vi "Remap Controls.vi"   [LabVIEW 2015]
uses:
  Common Code/Driver Control Selector.ctl
  Common Code/Manipulator Control Selector.ctl
  <vilib>/Rock Robotics/WPI/Utilities/WPI_GetSetVariantRefNum.vi
  Robot Global Data.vi
types:
  T1 = typedef "Manipulator Control Selector.ctl" = enum16{"High Pressure Shot", "Manual Climb Mode", "Auto Climb Mode", "Eject", "Intake", "Manual/Auto Toggle", "Re-seat", "Intake Down", "None"}
  T2 = typedef "Driver Control Selector.ctl" = enum16{"Creep Up", "Creep Down", "Creep Left", "Creep Right", "Forward/Backward", "Right/Left", "Outer Shot", "Batter Shot", "Shoot", "Climb", "Flashlight", "None"}
  T3 = typedef "Manipulator Control Remap.ctl" = cluster{"High Pressure Shot (B)":bool, "Manual Climb Mode (B)":bool, "Auto Climb Mode (B)":bool, "Eject (B)":bool, "Intake (B)":bool, "Manual/Auto (B) Toggle":bool, "Re-seat (A)":bool, "Intake Down (A)":bool}
  T4 = typedef "Driver Control Remap.ctl" = cluster{"Creep Up (P)":bool, "Creep Down (P)":bool, "Creep Left (P)":bool, "Creep Right (P)":bool, "Forward/Backward (A)":bool, "Right/Left (A)":bool, "Outer Shot (B)":bool, "Batter Shot (B)":bool, "Shoot (B)":bool, "Climb (B)":bool, "Flashlight (B)":bool}
  T5 = typedef "WPI_JoystickDevRef.ctl" = cluster{"Device":T6}
  T6 = typedef "WPI_JoystickDeviceEnum.ctl" = enum16{"USB 0", "USB 1", "USB 2", "USB 3", "USB 4", "USB 5"}
  T7 = typedef "D-Pad.ctl" = cluster{"Top":bool, "Bottom":bool, "None":bool, "Right":bool, "Left":bool}
  T8 = typedef "Button Cluster.ctl" = cluster{"Buttons[0]":bool, "Buttons[1]":bool, "Buttons[2]":bool, "Buttons[3]":bool, "Buttons[4]":bool, "Buttons[5]":bool, "Buttons[6]":bool, "Buttons[7]":bool, "Buttons[8]":bool, "Buttons[9]":bool}
  T9 = typedef "Axes Cluster.ctl" = cluster{"Axes[0]":dbl, "Axes[1]":dbl, "Axes[2]":dbl, "Axes[3]":dbl, "Axes[4]":dbl, "Axes[5]":dbl, "Axes[6]":dbl, "Axes[7]":dbl, "Axes[8]":dbl}
  T10 = typedef "Manipulator Control Indexes.ctl" = cluster{"High Pressure Shot":dbl, "Manual Climb Mode":dbl, "Auto Climb Mode":dbl, "Eject":dbl, "Intake":dbl, "Manual/Auto Toggle":dbl, "Re-seat":dbl, "Intake Down":dbl}
  T11 = typedef "Driver Control Indexes.ctl" = cluster{"Creep Up":dbl, "Creep Down":dbl, "Creep Left":dbl, "Creep Right":dbl, "Forward/Backward":dbl, "Right/Left":dbl, "Outer Shot":dbl, "Batter Shot":dbl, "Shoot":dbl, "Climb":dbl, "Flash Light":dbl}
  T12 = typedef "Manipulator Control Label.ctl" = cluster{"High Pressure Shot":string, "Manual Climb Mode":string, "Auto Climb Mode":string, "Eject":string, "Intake":string, "Manual/Auto Toggle":string, "Re-seat":string, "Intake Down":string}
  T13 = typedef "Driver Control Label.ctl" = cluster{"Creep Up":string, "Creep Down":string, "Creep Left":string, "Creep Right":string, "Froward/Backward":string, "Right/Left":string, "Outer Shot":string, "Batter Shot":string, "Shoot":string, "Climb":string, "Flashlight":string}
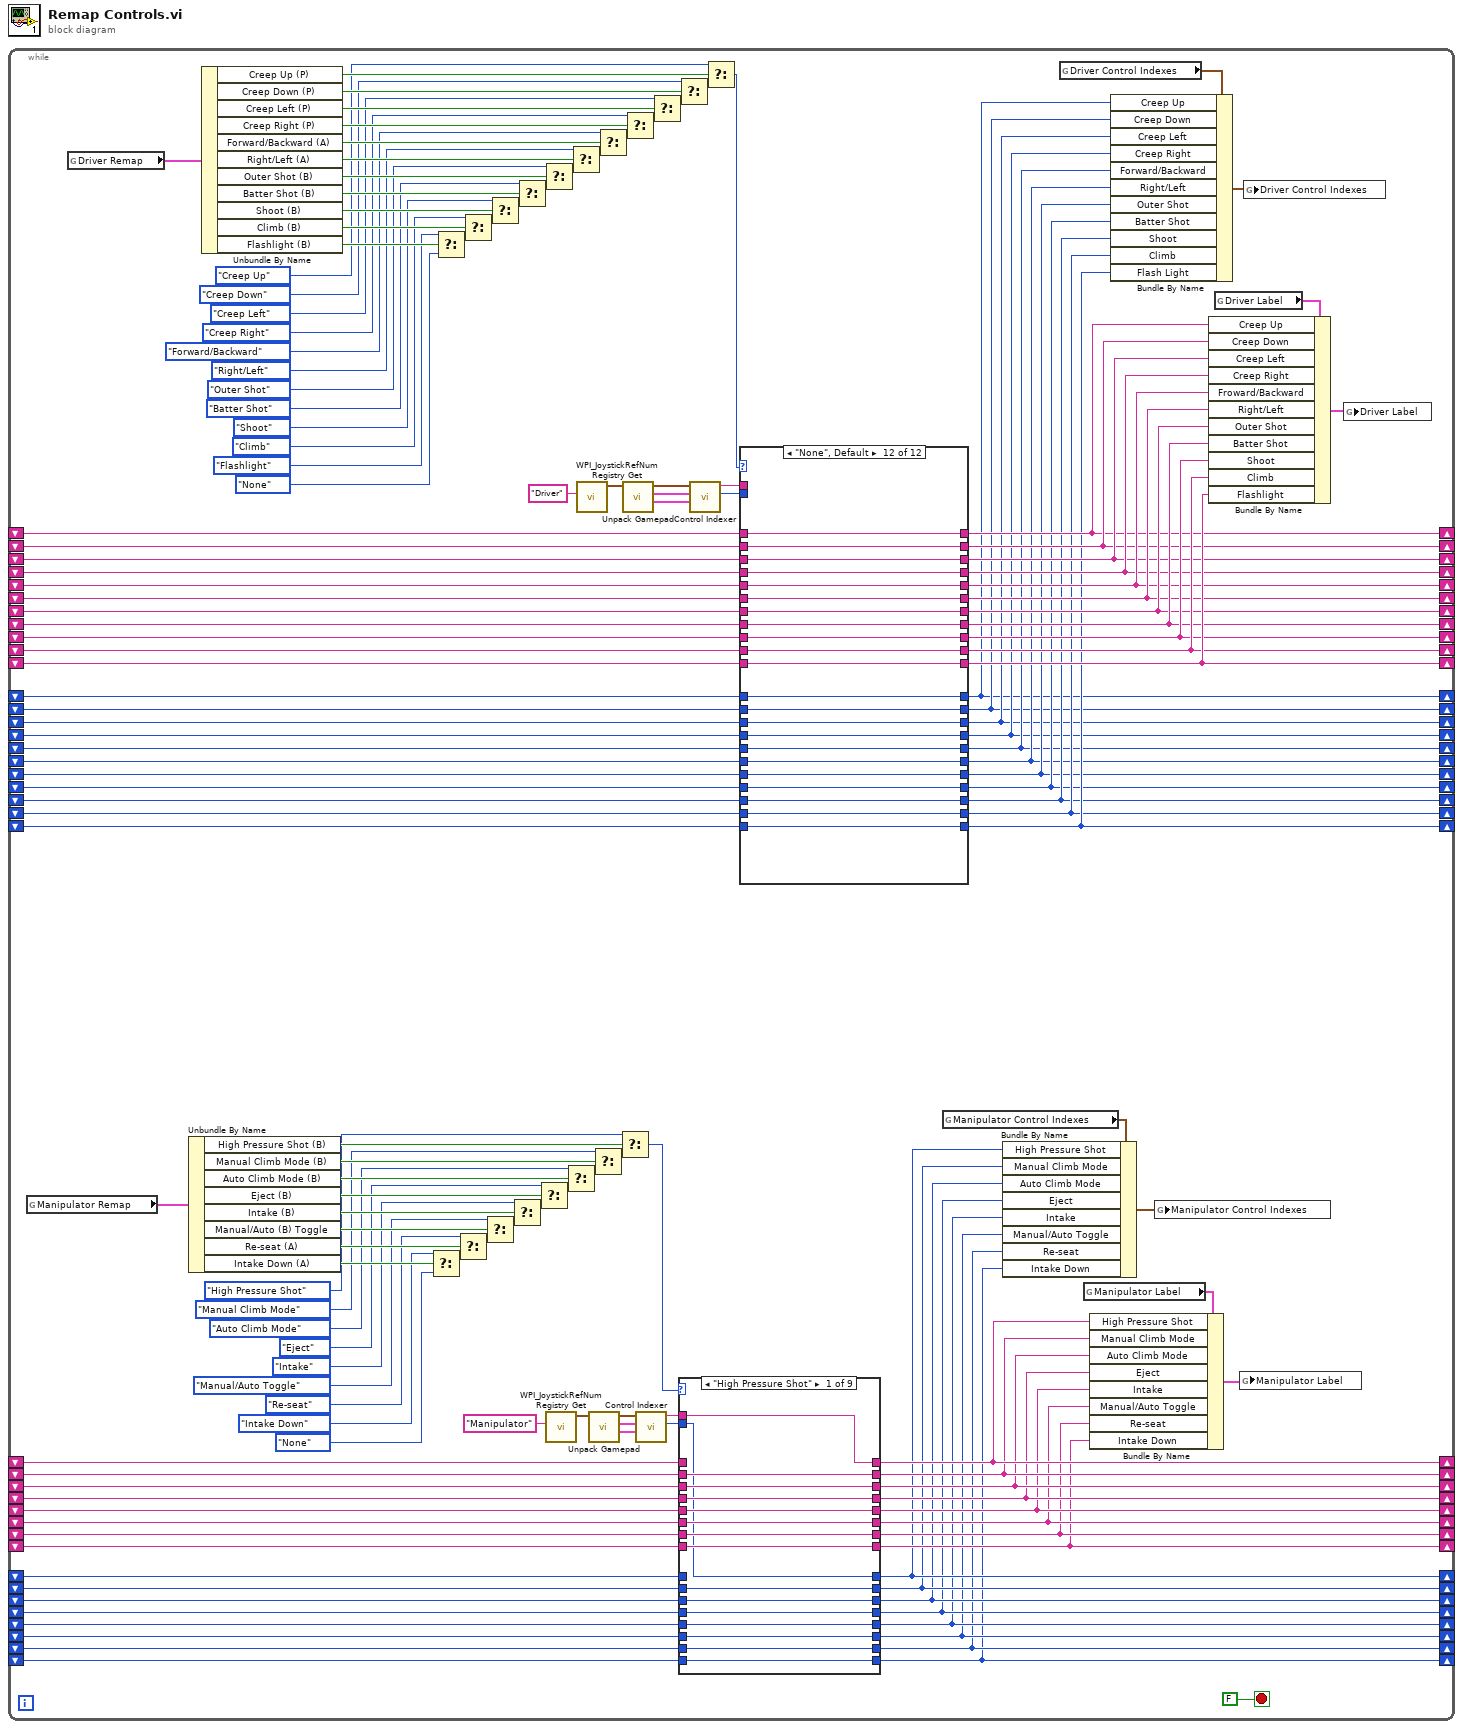
[diagram p0: block diagram]
diagram:
  n1 = while {
    shift-right: [w79] -> _
    shift-left: _ -> [w87]
    shift-right: [w78] -> _
    shift-left: _ -> [w86]
    shift-right: [w76] -> _
    shift-left: _ -> [w83]
    shift-right: [w77] -> _
    shift-left: _ -> [w85]
    shift-right: [w75] -> _
    shift-left: _ -> [w82]
    shift-right: [w74] -> _
    shift-left: _ -> [w84]
    shift-right: [w80] -> _
    shift-left: _ -> [w88]
    shift-right: [w81] -> _
    shift-left: _ -> [w91]
    shift-right: [w59] -> _
    shift-left: _ -> [w68]
    shift-right: [w58] -> _
    shift-left: _ -> [w67]
    shift-right: [w56] -> _
    shift-left: _ -> [w65]
    shift-right: [w57] -> _
    shift-left: _ -> [w66]
    shift-right: [w55] -> _
    shift-left: _ -> [w64]
    shift-right: [w54] -> _
    shift-left: _ -> [w63]
    shift-right: [w60] -> _
    shift-left: _ -> [w69]
    shift-right: [w61] -> _
    shift-left: _ -> [w70]
    shift-right: [w14] -> _
    shift-left: _ -> [w48]
    shift-right: [w15] -> _
    shift-left: _ -> [w47]
    shift-right: [w17] -> _
    shift-left: _ -> [w45]
    shift-right: [w16] -> _
    shift-left: _ -> [w46]
    shift-right: [w18] -> _
    shift-left: _ -> [w44]
    shift-right: [w19] -> _
    shift-left: _ -> [w43]
    shift-right: [w13] -> _
    shift-left: _ -> [w49]
    shift-right: [w12] -> _
    shift-left: _ -> [w50]
    shift-right: [w22] -> _
    shift-left: _ -> [w40]
    shift-right: [w21] -> _
    shift-left: _ -> [w41]
    shift-right: [w20] -> _
    shift-left: _ -> [w42]
    shift-right: [w3] -> _
    shift-left: _ -> [w37]
    shift-right: [w4] -> _
    shift-left: _ -> [w35]
    shift-right: [w6] -> _
    shift-left: _ -> [w34]
    shift-right: [w5] -> _
    shift-left: _ -> [w36]
    shift-right: [w7] -> _
    shift-left: _ -> [w33]
    shift-right: [w8] -> _
    shift-left: _ -> [w32]
    shift-right: [w2] -> _
    shift-left: _ -> [w38]
    shift-right: [w1] -> _
    shift-left: _ -> [w39]
    shift-right: [w11] -> _
    shift-left: _ -> [w29]
    shift-right: [w10] -> _
    shift-left: _ -> [w30]
    shift-right: [w9] -> _
    shift-left: _ -> [w31]
    stop <- FALSE stop-if-true
    n2 = global read "Robot Global Data.vi" "Manipulator Remap"() -> (w125:T3)
    n3 = global read "Robot Global Data.vi" "Driver Remap"() -> (w137:T4)
    n4 = Unbundle By Name(w125) -> ("High Pressure Shot (B)"=w124:bool, "Manual Climb Mode (B)"=w123:bool, "Auto Climb Mode (B)"=w117:bool, "Eject (B)"=w118:bool, "Intake (B)"=w119:bool, "Manual/Auto (B) Toggle"=w120:bool, "Re-seat (A)"=w121:bool, "Intake Down (A)"=w122:bool)
    n5 = Unbundle By Name(w137) -> ("Creep Up (P)"=w160:bool, "Creep Down (P)"=w159:bool, "Creep Left (P)"=w158:bool, "Creep Right (P)"=w157:bool, "Forward/Backward (A)"=w156:bool, "Right/Left (A)"=w155:bool, "Outer Shot (B)"=w154:bool, "Batter Shot (B)"=w153:bool, "Shoot (B)"=w152:bool, "Climb (B)"=w151:bool, "Flashlight (B)"=w150:bool)
    n6 = Select(t=Manipulator_Control_Selector."Intake Down", s=w122, f=Manipulator_Control_Selector."None") -> (s? t:f=w116:T1)
    n7 = Select(t=Driver_Control_Selector."Flashlight", s=w150, f=Driver_Control_Selector."None") -> (s? t:f=w139:T2)
    n8 = Select(t=Manipulator_Control_Selector."Re-seat", s=w121, f=w116) -> (s? t:f=w115:T1)
    n9 = Select(t=Driver_Control_Selector."Climb", s=w151, f=w139) -> (s? t:f=w140:T2)
    n10 = Select(t=Manipulator_Control_Selector."Manual/Auto Toggle", s=w120, f=w115) -> (s? t:f=w114:T1)
    n11 = Select(t=Driver_Control_Selector."Shoot", s=w152, f=w140) -> (s? t:f=w141:T2)
    n12 = Select(t=Manipulator_Control_Selector."Intake", s=w119, f=w114) -> (s? t:f=w113:T1)
    n13 = Select(t=Driver_Control_Selector."Batter Shot", s=w153, f=w141) -> (s? t:f=w142:T2)
    n14 = Select(t=Manipulator_Control_Selector."Eject", s=w118, f=w113) -> (s? t:f=w112:T1)
    n15 = Select(t=Driver_Control_Selector."Outer Shot", s=w154, f=w142) -> (s? t:f=w143:T2)
    n16 = call <vilib>:"WPI_JoystickRefNum Registry Get.vi"("refnum name"="Manipulator") -> ("JoystickDevRef"=w96:T5)  [unwired: 9 in, 1 out]
    n17 = Select(t=Manipulator_Control_Selector."Auto Climb Mode", s=w117, f=w112) -> (s? t:f=w111:T1)
    n18 = Select(t=Driver_Control_Selector."Right/Left", s=w155, f=w143) -> (s? t:f=w144:T2)
    n19 = call <vilib>:"WPI_JoystickRefNum Registry Get.vi"("refnum name"="Driver") -> ("JoystickDevRef"=w97:T5)  [unwired: 9 in, 1 out]
    n20 = call "Unpack Gamepad.vi"("JoystickDevRef"=w96) -> ("D-Pad"=w92:T7, "Button Cluster"=w93:T8, "Axes"=w94:T9)  [unwired: 8 in]
    n21 = Select(t=Manipulator_Control_Selector."Manual Climb Mode", s=w123, f=w111) -> (s? t:f=w110:T1)
    n22 = Select(t=Driver_Control_Selector."Forward/Backward", s=w156, f=w144) -> (s? t:f=w145:T2)
    n23 = Select(t=Manipulator_Control_Selector."High Pressure Shot", s=w124, f=w110) -> (s? t:f=w100:T1)
    n24 = call "Unpack Gamepad.vi"("JoystickDevRef"=w97) -> ("D-Pad"=w51:T7, "Button Cluster"=w52:T8, "Axes"=w53:T9)  [unwired: 8 in]
    n25 = Select(t=Driver_Control_Selector."Creep Right", s=w157, f=w145) -> (s? t:f=w146:T2)
    n26 = call "Control Indexer.vi"("D-Pad"=w92, "Button Cluster"=w93, "Axes"=w94) -> ("Index"=w62:i32, "Control Label"=w73:string)  [unwired: 7 in]
    n27 = Select(t=Driver_Control_Selector."Creep Left", s=w158, f=w146) -> (s? t:f=w147:T2)
    n28 = Select(t=Driver_Control_Selector."Creep Down", s=w159, f=w147) -> (s? t:f=w148:T2)
    n29 = case shown="\"High Pressure Shot\"" w100 {
      tunnel: w91 -> [_ w192 w207 w223 w239 w255 w271 w287 w304]
      tunnel: [w176 w192 w207 w223 w239 w255 w271 w287 w304] -> w81
      tunnel: w88 -> [w175 _ w206 w222 w238 w254 w270 w286 w303]
      tunnel: w87 -> [w174 w190 _ w221 w237 w253 w269 w285 w302]
      tunnel: w86 -> [w173 w189 w205 _ w236 w252 w268 w284 w301]
      tunnel: w85 -> [w172 w188 w204 w220 _ w251 w267 w283 w300]
      tunnel: w84 -> [w169 w185 w201 w217 w233 w249 w265 _ w297]
      tunnel: w83 -> [w171 w187 w203 w219 w235 _ w266 w282 w299]
      tunnel: w82 -> [w170 w186 w202 w218 w234 w250 _ w281 w298]
      tunnel: [w175 w191 w206 w222 w238 w254 w270 w286 w303] -> w80
      tunnel: [w174 w190 w208 w221 w237 w253 w269 w285 w302] -> w79
      tunnel: [w173 w189 w205 w224 w236 w252 w268 w284 w301] -> w78
      tunnel: [w172 w188 w204 w220 w240 w251 w267 w283 w300] -> w77
      tunnel: [w171 w187 w203 w219 w235 w256 w266 w282 w299] -> w76
      tunnel: [w170 w186 w202 w218 w234 w250 w272 w281 w298] -> w75
      tunnel: [w169 w185 w201 w217 w233 w249 w265 w288 w297] -> w74
      tunnel: w73 -> [w176 w191 w208 w224 w240 w256 w272 w288 _]
      tunnel: w70 -> [_ w183 w199 w215 w231 w247 w263 w279 w296]
      tunnel: w69 -> [w167 _ w198 w214 w230 w246 w262 w278 w295]
      tunnel: w68 -> [w166 w182 _ w213 w229 w245 w261 w277 w294]
      tunnel: w67 -> [w165 w181 w197 _ w228 w244 w260 w276 w293]
      tunnel: w66 -> [w164 w180 w196 w212 _ w243 w259 w275 w292]
      tunnel: w65 -> [w163 w179 w195 w211 w227 _ w258 w274 w291]
      tunnel: w64 -> [w162 w178 w194 w210 w226 w242 _ w273 w290]
      tunnel: w63 -> [w161 w177 w193 w209 w225 w241 w257 _ w289]
      tunnel: w62 -> [w168 w184 w200 w216 w232 w248 w264 w280 _]
      tunnel: [w168 w183 w199 w215 w231 w247 w263 w279 w296] -> w61
      tunnel: [w167 w184 w198 w214 w230 w246 w262 w278 w295] -> w60
      tunnel: [w166 w182 w200 w213 w229 w245 w261 w277 w294] -> w59
      tunnel: [w165 w181 w197 w216 w228 w244 w260 w276 w293] -> w58
      tunnel: [w164 w180 w196 w212 w232 w243 w259 w275 w292] -> w57
      tunnel: [w163 w179 w195 w211 w227 w248 w258 w274 w291] -> w56
      tunnel: [w162 w178 w194 w210 w226 w242 w264 w273 w290] -> w55
      tunnel: [w161 w177 w193 w209 w225 w241 w257 w280 w289] -> w54
      frame "High Pressure Shot" {
      }
      frame "Manual Climb Mode" {
      }
      frame "Auto Climb Mode" {
      }
      frame "Eject" {
      }
      frame "Intake" {
      }
      frame "Manual/Auto Toggle" {
      }
      frame "Re-seat" {
      }
      frame "Intake Down" {
      }
      frame "None", Default {
      }
    }
    n30 = call "Control Indexer.vi"("D-Pad"=w51, "Button Cluster"=w52, "Axes"=w53) -> ("Index"=w27:i32, "Control Label"=w28:string)  [unwired: 7 in]
    n31 = Select(t=Driver_Control_Selector."Creep Up", s=w160, f=w148) -> (s? t:f=w138:T2)
    n32 = case shown="\"None\", Default" w138 {
      tunnel: w50 -> [_ w346 w368 w390 w407 w435 w456 w478 w500 w523 w545 w568]
      tunnel: w49 -> [w324 _ w367 w389 w406 w434 w455 w477 w499 w522 w544 w567]
      tunnel: w48 -> [w323 w345 _ w388 w405 w433 w454 w476 w498 w521 w543 w566]
      tunnel: w47 -> [w322 w344 w366 _ w404 w432 w453 w475 w497 w520 w542 w565]
      tunnel: w46 -> [w321 w343 w365 w387 _ w431 w452 w474 w496 w519 w541 w564]
      tunnel: w45 -> [w320 w342 w364 w386 w413 _ w451 w473 w495 w518 w540 w563]
      tunnel: w44 -> [w319 w341 w363 w385 w412 w430 _ w472 w494 w517 w539 w562]
      tunnel: w43 -> [w318 w340 w362 w384 w411 w429 w450 _ w493 w516 w538 w561]
      tunnel: w42 -> [w317 w339 w361 w383 w410 w428 w449 w471 _ w515 w537 w560]
      tunnel: w41 -> [w316 w338 w360 w382 w409 w427 w448 w470 w492 _ w536 w559]
      tunnel: w40 -> [w315 w337 w359 w381 w408 w426 w447 w469 w491 w514 _ w558]
      tunnel: w39 -> [_ w336 w358 w380 w402 w424 w446 w468 w490 w513 w535 w557]
      tunnel: w38 -> [w314 _ w357 w379 w401 w423 w445 w467 w489 w512 w534 w556]
      tunnel: w37 -> [w313 w335 _ w378 w400 w422 w444 w466 w488 w511 w533 w555]
      tunnel: w36 -> [w311 w333 w355 w377 _ w420 w442 w464 w486 w509 w531 w553]
      tunnel: w35 -> [w312 w334 w356 _ w399 w421 w443 w465 w487 w510 w532 w554]
      tunnel: w34 -> [w310 w332 w354 w376 w398 _ w441 w463 w485 w508 w530 w552]
      tunnel: w33 -> [w309 w331 w353 w375 w397 w419 _ w462 w484 w507 w529 w551]
      tunnel: w32 -> [w308 w330 w352 w374 w396 w418 w440 _ w483 w506 w528 w550]
      tunnel: w31 -> [w307 w329 w351 w373 w395 w417 w439 w461 _ w505 w526 w549]
      tunnel: w30 -> [w306 w328 w350 w372 w394 w416 w438 w460 w482 _ w527 w548]
      tunnel: w29 -> [w305 w327 w349 w371 w393 w415 w437 w459 w481 w503 _ w547]
      tunnel: w28 -> [w326 w348 w370 w392 w414 w436 w458 w480 w502 w524 w546 _]
      tunnel: w27 -> [w325 w347 w369 w391 w403 w425 w457 w479 w501 w504 w525 _]
      tunnel: [w326 w346 w368 w390 w407 w435 w456 w478 w500 w523 w545 w568] -> w12
      tunnel: [w324 w348 w367 w389 w406 w434 w455 w477 w499 w522 w544 w567] -> w13
      tunnel: [w323 w345 w370 w388 w405 w433 w454 w476 w498 w521 w543 w566] -> w14
      tunnel: [w322 w344 w366 w392 w404 w432 w453 w475 w497 w520 w542 w565] -> w15
      tunnel: [w321 w343 w365 w387 w414 w431 w452 w474 w496 w519 w541 w564] -> w16
      tunnel: [w320 w342 w364 w386 w413 w436 w451 w473 w495 w518 w540 w563] -> w17
      tunnel: [w319 w341 w363 w385 w412 w430 w458 w472 w494 w517 w539 w562] -> w18
      tunnel: [w318 w340 w362 w384 w411 w429 w450 w480 w493 w516 w538 w561] -> w19
      tunnel: [w317 w339 w361 w383 w410 w428 w449 w471 w502 w515 w537 w560] -> w20
      tunnel: [w316 w338 w360 w382 w409 w427 w448 w470 w492 w524 w536 w559] -> w21
      tunnel: [w315 w337 w359 w381 w408 w426 w447 w469 w491 w514 w546 w558] -> w22
      tunnel: [w325 w336 w358 w380 w402 w424 w446 w468 w490 w513 w535 w557] -> w1
      tunnel: [w314 w347 w357 w379 w401 w423 w445 w467 w489 w512 w534 w556] -> w2
      tunnel: [w313 w335 w369 w378 w400 w422 w444 w466 w488 w511 w533 w555] -> w3
      tunnel: [w312 w334 w356 w391 w399 w421 w443 w465 w487 w510 w532 w554] -> w4
      tunnel: [w311 w333 w355 w377 w403 w420 w442 w464 w486 w509 w531 w553] -> w5
      tunnel: [w310 w332 w354 w376 w398 w425 w441 w463 w485 w508 w530 w552] -> w6
      tunnel: [w309 w331 w353 w375 w397 w419 w457 w462 w484 w507 w529 w551] -> w7
      tunnel: [w308 w330 w352 w374 w396 w418 w440 w479 w483 w506 w528 w550] -> w8
      tunnel: [w307 w329 w351 w373 w395 w417 w439 w461 w501 w505 w526 w549] -> w9
      tunnel: [w306 w328 w350 w372 w394 w416 w438 w460 w482 w504 w527 w548] -> w10
      tunnel: [w305 w327 w349 w371 w393 w415 w437 w459 w481 w503 w525 w547] -> w11
      frame "Creep Up" {
      }
      frame "Creep Down" {
      }
      frame "Creep Left" {
      }
      frame "Creep Right" {
      }
      frame "Forward/Backward" {
      }
      frame "Right/Left" {
      }
      frame "Outer Shot" {
      }
      frame "Batter Shot" {
      }
      frame "Shoot" {
      }
      frame "Climb" {
      }
      frame "Flashlight" {
      }
      frame "None", Default {
      }
    }
    n33 = global read "Robot Global Data.vi" "Manipulator Control Indexes"() -> (w72:T10)
    n34 = Bundle By Name(cluster=w72, "High Pressure Shot"=w61, "Manual Climb Mode"=w60, "Auto Climb Mode"=w59, "Eject"=w58, "Intake"=w57, "Manual/Auto Toggle"=w56, "Re-seat"=w55, "Intake Down"=w54) -> (w71:T10)
    n35 = global read "Robot Global Data.vi" "Driver Control Indexes"() -> (w24:T11)
    n36 = global read "Robot Global Data.vi" "Manipulator Label"() -> (w90:T12)
    n37 = Bundle By Name(cluster=w90, "High Pressure Shot"=w81, "Manual Climb Mode"=w80, "Auto Climb Mode"=w79, "Eject"=w78, "Intake"=w77, "Manual/Auto Toggle"=w76, "Re-seat"=w75, "Intake Down"=w74) -> (w89:T12)
    n38 = Bundle By Name(cluster=w24, "Creep Up"=w1, "Creep Down"=w2, "Creep Left"=w3, "Creep Right"=w4, "Forward/Backward"=w5, "Right/Left"=w6, "Outer Shot"=w7, "Batter Shot"=w8, "Shoot"=w9, "Climb"=w10, "Flash Light"=w11) -> (w23:T11)
    n39 = global write "Robot Global Data.vi" "Manipulator Control Indexes"(w71) -> ()
    n40 = global read "Robot Global Data.vi" "Driver Label"() -> (w26:T13)
    n41 = Bundle By Name(cluster=w26, "Creep Up"=w12, "Creep Down"=w13, "Creep Left"=w14, "Creep Right"=w15, "Froward/Backward"=w16, "Right/Left"=w17, "Outer Shot"=w18, "Batter Shot"=w19, "Shoot"=w20, "Climb"=w21, "Flashlight"=w22) -> (w25:T13)
    n42 = global write "Robot Global Data.vi" "Manipulator Label"(w89) -> ()
    n43 = global write "Robot Global Data.vi" "Driver Control Indexes"(w23) -> ()
    n44 = global write "Robot Global Data.vi" "Driver Label"(w25) -> ()
  }
